vi "singleActionGUI.vi"() -> ()   [LabVIEW 2013]
panel:
  in  "VISA resource":refnum<visa-resource-name>="COM3"
  in  "Stop VI":bool
  out "Max speed (mm):   2":dbl=18.0 format="%#.3g"
  out "Step size (mm):   2":dbl=0.49609375 format="%#.3g"
  out "Max position (mm):  2":dbl=151.49760546875 format="%#.3g"
  out "Current position (mm): 2":dbl format="%#.3g"
  in  "Position (mm) 2":dbl min=-151.488 max=151.498 step=0.001 format="%#.3g"
  in  "right but":bool
  in  "left but":bool
  in  "go but":bool
  in  "home but":bool
  in  "stop but":bool
  in  "radio but":enum32{"Absolute", "Relative"}(radio)
  in  "Speed (mm/s) 2":dbl=13.59 min=0.1 max=18.0 step=0.001 format="%.3g"
  in  "?":bool
  in  "?":bool
  out "Max speed (mm/s):":dbl
  in  "?":dbl
  out "Max extension (mm):":dbl
  out "Current position (mm):":dbl
  out "Max force (N):":dbl
  out "Current force (N):":dbl
  in  "?":dbl
  in  "?":bool
  in  "?":bool
  in  "?":bool
  in  "?":enum32{"", ""}(radio)
  # "Stage panel"
  # "Roller panel"
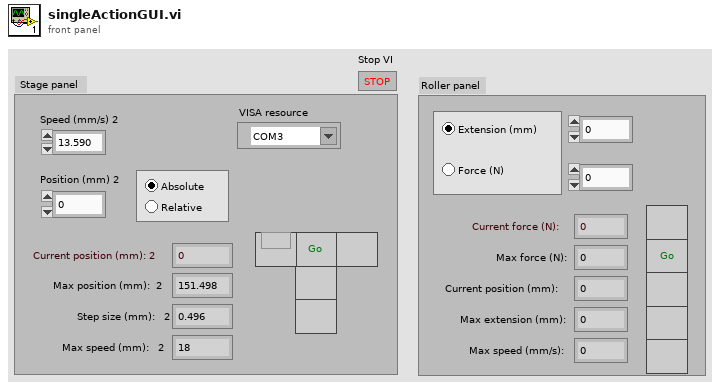
[diagram p1: front panel]
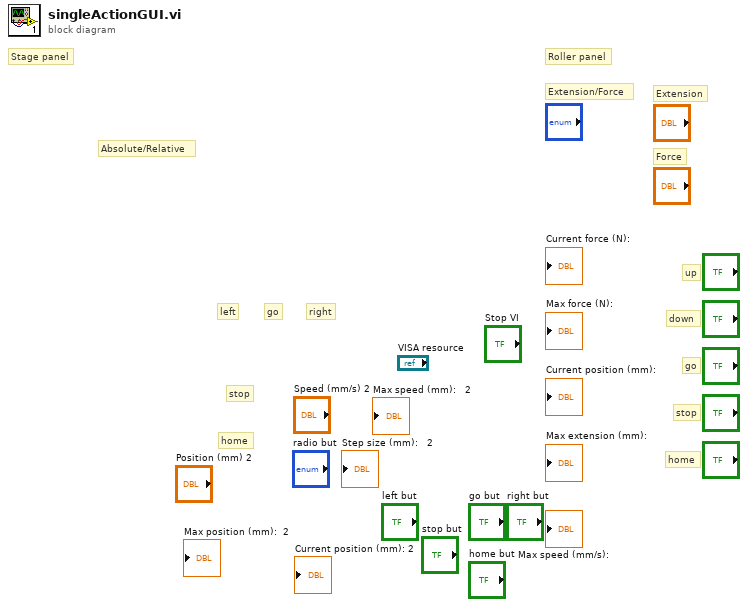
[diagram p0: block diagram]
diagram:
  # "Force"
  # "Extension"
  # "Extension/Force"
  # "Absolute/Relative"
  # "home"
  # "stop"
  # "right"
  # "left"
  # "go"
  # "home"
  # "stop"
  # "go"
  # "down"
  # "up"
  # "Roller panel"
  # "Stage panel"
